vi "Main_12b.vi"() -> ()   [LabVIEW 2023]
uses:
  ENUM_Type.ctl
  <vilib>/Utility/error.llb/Trim Whitespace One-Sided.vi
panel:
  out "container size":i32
  out "appended array":T1[](array[typedef])
  out "Function Array min size":i32
  out "Array":cluster{"Array":T1[]}[](array[cluster])
  out "Rows Left":i32
  out "Complete Match Count":i32
  in  "Enum":T1
  out "Answer":i32
  in  "Puzzle":string="??#.????#???.#?# 1,5,1,1,1\n?##?##??#? 7,1\n??????#???. 1,7\n??#?#??#.?#.??#? 5,1,1,2\n???????.??? 1,3\n?#..##?##??###??#? 2,13\n?.????????.???????? 1,5,1,6\n?.???#???. 2,2\n??#..#???#? 1,1,4\n?.?##?????#??? 1,5,2,1\n.???#?????##??#.? 3,8\n?????????????.#.. 4,3,1\n..#???????.? 4,3,1\n????#??.?.#??? 7,3\n#??#???##??.?? 4,1,3,2\n??#?#?##?.???#??. 6,5\n???.#??.??###?.#?? 3,1,5,2\n?.????##??#?? 6,3\n???..?##????.? 2,3,1\n?.?#????.??#?#.? 1,2,1,3,1\n?.?###.???? 4,2\n?#???..??##? 4,3\n???#????#?. 1,2,3\n#???#???#??#???.? 1,10,1\n???????????????????? 1,5,6,3\n???????#??? 2,6\n??.??.????.?#?????# 1,1,2,1,4,3\n???#???.??#? 1,4,1,1\n???#???##??##? 3,2,3\n????.??????#?.#? 1,1,1,4,2\n?.#??#???? 1,1,5\n??##???#?.##??..? 4,2,4\n??????#.????.# 4,2,1,1\n??????#??#?.??? 2,7,1\n.????????##.?.?.##? 5,2,1,1,2\n.??????????#?#. 3,1,2,1\n?????????????. 2,1,5\n?##????#?.?????.#??? 2,1,2,3,3\n?????????#?.?????#? 1,2,1,3,4,2\n..?.#???.?##.? 1,3,2\n.??????????????? 10,2\n?.?#????#?.??? 1,1,2,2\n??????.#??.?.? 1,1,1\n#???#?#??#????? 1,2,1,5\n???.?.??#????.? 3,6\n.#.???###???.#?..??? 1,8,2,2\n.???.??#????# 2,4,1\n.????#?#?? 3,3,1\n?###??#??## 4,2,2\n??#?#???#???.??. 3,5,1\n???####??##..?#.#.?? 9,2,1,1\n??#?#???#.?. 5,1\n???#????#???##?# 2,3,3,1\n?#???????#???#??? 1,3,3,3,1\n#???#????#.##..? 8,1,2\n?????.?#?#??? 1,5\n.??#.??#?.? 1,1,1\n?#?#???#???.??? 1,1,4,1,3\n.????#.?.#??? 1,1,2,1\n.??#?.??#? 4,2\n#????????. 1,4,1\n??.#?#????#?...?? 1,8,2\n?#.#?#.??##? 2,3,1,2\n...??.?#?? 1,1\n?.?.????#..? 1,2,1\n?##????????.??.?#??? 6,1,1,4\n?.??#.??.?.???? 3,2\n.????.?????.???.?? 4,1,1,3,1\n?????????##???????#? 2,1,1,2,2,2\n???.?????.????? 2,3,5\n???#??????.??#??.? 1,6,1,1,1\n??##??????###??? 12,1\n?.??.?????? 1,1,2\n??#??????#?.. 2,5\n???#####????. 1,8\n.?#?##??????#??.???? 6,2,1\n?.#??#???????#????? 1,1,12,1\n??????????#.?..?##? 1,1,1,1,3,3\n???????#???.??## 10,4\n.?#????.?.???..? 1,1,2\n.???#?#????? 2,2,1\n#????#?.????##?#?# 1,5,1,5,1\n???.##??????##??#? 1,2,8,2\n??#????????????#? 6,7\n????.??.#.?#?#? 1,1,1,1,4\n??##?#??.#???? 6,1,4\n?#?.?#????????#?. 3,2,4,3\n..??????##?# 2,1,2,1\n?????????.???? 4,1,1,1\n.??#?????.?.?. 1,6,1\n#.?#?#??????#??# 1,6,2,1,1\n.#?.#.##??# 1,1,5\n??#?????#?????? 5,4\n.#??.?.?.? 2,1\n.?#???##.????##?? 7,2\n?#?.??????#??????# 1,8,3\n?.#??#??.?#.. 4,1,1\n?#?#?#??????? 7,1,1\n?#???????? 6,1\n????#..?#???##? 1,1,2,3\n..?????#?###??.? 1,9,1\n?##???.???#?# 4,4\n??.??#???..??#? 1,2,1,3\n#?#??????.??#?? 8,1,3\n???#?##?#?? 2,6\n.?.???#???.#?????? 1,3,1,5,1\n?#.???????# 2,2,1\n?.???.??.? 1,1,1\n?#?#?#??????#??#??? 1,5,2,4,2\n?#??.?#?????.?#. 4,6,2\n#???.?#?#??#?.??#? 2,7,1\n.??#...???????. 3,1,1\n?..???##??. 1,6\n??#??#?#??? 2,4\n?.?.??.??????#?. 1,7\n?.?????????.??. 2,2,2\n???.?????? 2,1\n???.??????????? 1,3,4,1\n?#????#???#??? 10,1\n??#???.?????#???# 6,3,1\n????.?##??#??# 3,8\n?????????????. 1,7,1\n?..?????.#???.. 1,4,2\n?.???#???#? 1,5,1\n#???.????? 2,1,1\n?#.??#?.???? 1,1,1,1\n????.?#???.???. 1,1,4,2\n.?#??#??.??????? 2,4,6\n.??.?##.??#?#.??? 2,3,2,1,1\n..??????#?.?? 2,2\n???#?#??.##. 3,2,2\n?..?????????##?#??? 1,13,1\n??#?????#?.??#?????? 6,2,5,2\n???.???#???# 1,1,3,1\n??##????.?. 4,1\n??#??#??#?. 3,6\n.??????#????#.#.?? 1,1,8,1,1\n?#?#?.?.?.###??#???? 5,1,1,3,1,1\n???.#?#???.?? 1,1,5,1\n?????####??????? 2,5,2,1\n????.??#??#? 1,1,2,1\n??.?????#?#.????? 2,3,3\n?#??#?#?.????.??? 2,3,2,2\n?????????#??.??????. 1,6,1,1,1,1\n???.##?##??#? 1,6,1\n????#?.??.. 4,1\n?#??#?#???.????#?# 4,4,6\n?????#??#.#? 1,2,2,1\n?#?#?#??###??? 1,1,7\n.##?.????? 3,3\n??#???###????? 1,6\n.?###????????##?#?? 7,1,5\n..?#????????#? 3,5\n#?#???.??? 1,1,1\n#???????????#??.??? 10,3,1\n???##??#??#?.?????. 10,3\n?#?????.???????## 3,2,5,3\n??.??#####???. 2,8\n???.?????? 1,1,3\n???#???????????. 6,4\n#???#?????##???.?#? 2,1,1,5,2\n?#?..???#??????. 2,7,2\n?????##?#? 2,3,2\n.#?..????# 2,3\n???????#??#.?..??.. 3,1,1,2,1,1\n?.#??#????? 1,3,2\n???..?.?.? 1,1,1\n?#.?#??#???.##.? 1,1,4,2\n???#?#.??#??? 4,1\n??????#????.???? 6,1,1,1,2\n???..??.#???? 1,1,1,2\n????????.? 1,1,1\n?..#??.??. 3,1\n?##.??#??? 2,1,1\n?????#?????#?#?? 2,12\n?#??????#???.?? 1,6,2,1\n#??.???.??##???.#? 2,3,7,2\n???????..????#????? 2,1,1,7,1\n????#??.?????? 1,2,4\n?###?#?##?##??.??. 12,1\n?#??#.?.??#?... 3,1,1,1,2\n??#??#??#????#? 9,2\n???????##????? 1,1,5\n?.?#????#?.??.?? 3,3,1,1\n???..??????#..??#? 1,1,7,1,1\n??.???###???#..? 1,1,5,1,1\n??.??.#????#????# 2,1,7,2\n??????#?#??????# 1,6,1\n#?.?...??.??????? 1,1,1,6\n??#?##??#?..## 7,2\n?#?###..?.#?##??.?.# 5,6,1\n.??.?.???. 2,1,1\n?.???..?.?#?.??.???? 1,3\n.#?.??????.?.?#??? 2,6,4\n???##...??. 3,1\n????????????#?????. 4,6\n????#.??#? 1,1,1\n?.?#.??..??#?????..? 1,2,1,8\n?????.??.? 1,2,1\n??????##?.?? 1,4\n???.????#??? 1,1,5\n.??#???.#.#??#??. 6,1,2,1,1\n?.????#??##?????? 1,1,1,7\n??????##.??? 3,2,1\n?.????#?????.?.? 1,4,2,1\n?????????????## 1,1,2,4\n.?##??#??.??# 4,1,3\n??#?##??#?? 2,5,1\n?????.###??.?.#??# 1,1,4,1,1,1\n.????????##?#? 1,7\n??????????.? 7,1\n.?????###????..#. 12,1\n????.????? 3,1,1\n#.??#????#????#????? 1,5,1,7,1\n.##??????.??##? 7,3\n?..?.???#?????###? 1,1,5,5\n??????#???. 1,1,3\n??.#???????##????. 1,2,3,6\n?.?.?.?.#???????#?. 1,1,1,1,2,7\n?????#????????. 1,1,1,4,1\n?.??#??#?? 1,1,2\n??#???.#.?#?#?? 1,1,1,1,5\n?????????.? 4,1\n??.?????#?.?.#?? 7,1\n??.?#.?????#??. 2,7\n?????##..? 1,4\n?????????. 4,1\n??.?..?#???? 2,3,2\n????.####??###? 2,4,4\n?####???##??????? 10,1,1\n???#?#???# 1,5,1\n????###.??.?????#??. 6,1,6\n#???????#?. 2,1,4\n?#?.???##???????#? 3,1,2,1,6\n???#??#?.?.?????? 1,5,1,1,4\n?.#???##???.?.## 1,3,2,2\n???..##?.?.? 2,2,1\n?.#?#?????. 3,1\n????.##?#?#??##?? 3,12\n#?##???????? 1,3,3,1\n???.#?.????##? 1,2,1,4\n???.??#???? 1,3\n.???###??.???????# 7,5,1\n?#.??.?#???##?. 1,1,1,4\n.????###????? 2,6\n???#???.???????#?? 1,2,1,3,4,1\n.?.?????????? 3,5\n??#???#?.###????.?? 7,3,1,1,1\n#??###??#?#.????? 11,1\n#.?????#??#.##???.? 1,1,7,5\n??????.????#???? 1,1,4,1,1\n?.?#?#?#??###?? 7,4\n????#???#?#?###????? 1,2,10,1\n????#????? 1,4,2\n???.#??#????.?#??.?. 3,2,1,1,4,1\n?????.?#??????. 1,2,1,1,1\n?#???????#?#?#???.? 2,12\n?#??..??.???###?? 4,2,1,5\n##????????#.? 5,2\n#?#?.?.??###??#?. 4,8\n??##?.???? 3,4\n?.????##???????? 8,1,1\n#????#??#???#?#.??? 15,1\n?.?????.#? 4,2\n?.##???..?? 1,3,1\n#????#??????????#?? 2,7,2,3\n???.????#? 1,1,2\n??..#?????### 1,3\n????????.?? 2,4,1\n#??##??#.?????.??? 1,5,2,1,1,1\n???#.?#?#?. 3,1,2\n?##?#??????#?#.# 3,3,3,1,1\n??.#?..??? 1,1,1\n?#??.???#? 1,1,3\n???#???????.??##?? 8,3\n??.#.?#???#??.? 2,1,7\n??????.####?.?#?# 4,4,4\n??????????? 2,2,1\n?#?.??.???.? 2,2\n????#?#?## 6,2\n.??###??????.? 5,3\n.???#.#????? 3,5\n?##?#?.?#?#??. 6,2,1,1\n#.???.??#?####?..? 1,1,1,8,1\n????#???#???# 1,1,2,3\n?????.??.#???#? 3,5\n?#??..?????????#?. 1,1,3,1,4\n#?????????????.?? 6,1,1,1\n?#?????..?????#??# 3,1,1,5\n???????.???????????? 1,4,1,9\n.????????????.. 2,1,6\n.?#??????. 2,4\n??#??#???#.???#? 1,5,2,1,2\n.?.???????.?.#??? 4,1,2\n##?.??##?..???. 3,4,3\n??..??#??#?. 1,6\n??#??????????##???? 2,6,4,1\n??..????##?????? 1,5\n##????????.??.#??? 2,6,4\n?#??#...?????# 2,2,1,2\n?..??????.???.?# 1,1,3,1,1\n.?###??#???#???? 7,4,1\n?#?.?????. 2,2\n??..????.?????# 1,1,2,2\n??##.#??????.##??#?? 1,2,1,1,1,5\n??.##??????#???#??? 4,8\n??#?????????. 4,3,2\n#????.???? 1,1,1\n?..??.?????? 2,3\n??????#??###???? 1,1,9,1\n?????#?#???????.. 1,6,3\n?#??.???#?##. 3,3,2\n?..##?#???????#?? 9,1\n???.?#?#?#?. 1,5\n???##?#???#?# 8,3\n?##??#??.??.???????? 2,3,1,6\n.??...?????????#.#? 1,6,2,2\n????.#??#?#.##?. 1,1,1,3,3\n?#?#?????.??????. 5,3\n??.????##???. 1,5\n????#?.???? 2,1\n????..??#???. 4,2,1\n???????.?# 2,1\n????????????? 1,1,3\n???##??????###.?#? 2,2,2,3,1\n??????#?#?#?#?## 3,10\n?????#??..????????? 8,5\n??##???????.??? 6,1,1,2\n?.???.????.??? 3,1,1,3\n.?.???.??? 1,2\n.???###???#??.?? 5,1,1,1\n????#?.##?###.# 1,3,2,3,1\n.?#???????? 1,4\n?#?#?????????### 8,6\n?????..???.???? 4,3,1,1\n..?#?.?#??? 1,5\n.????.??#? 3,3\n?##????.?#??????..?? 7,3,3,1\n?????##??.?.??...?? 9,2,2\n??..#??####??.?.?#? 8,2\n??????##????? 1,1,6\n??????#??.???#? 7,5\n???#..??.????. 4,1,2\n.#?.?###??? 1,4\n????###?...?#?#? 8,4\n?????#???#??????? 1,1,6,1,1\n.??#?#?##??????? 7,1,1\n.#.?????#.?#### 1,2,1,1,5\n?#??..#??.#?? 3,1,1,1\n????#??.???. 3,1,3\n#.???#???. 1,2\n???.???##.???.? 1,1,2,2\n?#?#..?#????##?.?. 3,9\n.?.??.????? 2,2\n??????.?.##?#?.? 5,4\n???#???.????? 7,1\n??####?????.???#?? 6,3,4\n?.?...?#.#?#??? 1,2,5\n??.??#??#?#?#??.?? 2,3,7,1\n?#?.???????? 1,1,1\n????????#?##?#??? 1,2,9,1\n#???.???#????.??#??? 3,1,1,1,4,1\n.??#?.?.#??? 2,1,2,1\n.?##?###.###?#?.??. 6,5,2\n.?.???????#????##? 3,10\n?.##???..#? 5,2\n????????????#??.???? 1,1,10,1\n??##??#.??#??#?? 5,3,2,1\n?#???#.??????..# 6,4,1,1\n????????.? 1,2,2\n?????#??#??#????#??? 14,2,1\n???#??.???#?#???? 4,7,1\n.?.##?.???#??..????? 1,3,4,2\n??????#??????? 1,1\n..#?##??.????. 5,3\n??????????#.? 4,1\n#????.???.? 1,1\n.?..?#.??? 2,1\n?#.??##??.##?.?? 2,4,2,2\n??#????#??????? 9,1\n.#?.##?##.#???? 1,5,1,1\n?#?###???#??#?.??? 11,1,1\n???#??..?? 3,1\n#?#??????#?????#? 12,2\n??#?#?.???.? 2,2,3,1\n?#???.?.??#?#???? 5,1,8\n.???#?#??#?????. 10,1\n??????.?????.? 5,1,1,1\n.?.??????????# 3,7\n.#?.??..##??.?#..#? 1,1,4,2,1\n?##?#??.??###?????# 2,1,1,1,7,1\n?##?.???.? 2,1,1\n?????#.#?##.?#? 1,1,4,1\n?#?.??.?#.#.##.? 2,1,1,1,2\n???????.#.??##??.?. 6,1,3,1,1\n.?#??#???????#???.#. 3,1,1,2,4,1\n?????#?.##??##??.?? 1,2,2,3,2\n#??.???????? 1,1,1,1\n????#?.##?.?#?#?# 5,2,5\n.?.??.#?????????..?# 1,1,6,1,2\n???#?#?????. 7,2\n???????##??#?.?#?.? 1,8,3\n.?..?#?#???? 4,1\n??.?#??.????. 1,1,3\n????##???##???#??? 12,4\n?###?#??..#?.??? 6,1,2,1\n##??..##?#????# 3,2,1,1\n?????#?##??##???#?? 2,13\n#?..???##???##?#???? 2,6,4,1,1\n.????.?....#????. 1,3\n?.?.??#??#.?# 1,2,1,2\n???#??.??#.? 1,1,1,2\n.????#?#???#??????? 12,1,1\n?..#??#?##??#???? 1,1,2,3,5\n.#??##?##??????.?# 2,11,2\n.?.#?#?.?#???#.? 1,4,6\n?#.##??.????? 2,4,4\n???.??????.??. 2,1,1,2\n???????.?##.#???.? 1,1,1,2,3,1\n??..???????#?.? 5,2\n?????#????? 3,2,2\n.##????..#??.. 6,2\n????.??????.???###? 3,3,1,5\n??????#?.???# 1,3,1,1\n????#????. 6,1\n??.?#????. 1,4\n??????#???##???. 6,1,3,1\n?.?#.????. 1,1,4\n?##??.#?#??.#?? 3,1,1,1,1\n?.?#??????. 1,5,1\n???????#?. 1,4\n???#????#?##?#?????? 2,2,1,1,6,1\n??##.?????##??#.? 1,2,7,1\n????????.# 4,1\n.???#????? 1,1,1\n?.?#??.????.?#?? 1,4,2,2,1\n.?##?#???.??..?#? 3,3,3\n?#??.?.?#??? 1,1,4\n????..#????#.?? 1,1,1,3,2\n???#?..??? 5,1\n?##???##.?. 3,2,1\n??#???.???### 2,1,1,3\n????.?#??##?. 2,2,2\n?#???##??#?????#.??? 2,11,1\n???#??..?##??# 5,6\n????.??#???.#?#.?#?# 2,5,1,1,1,1\n?.??????#??? 2,3,2\n#.#???..????????. 1,1,2,6,1\n?.?..?.#??????##?? 1,1,1,1,3,5\n.??.?.???? 1,1,4\n#??#.?#?#???#??????# 1,1,2,1,1,8\n?????.?#..#. 3,1,1\n????##???.?????.. 5,3\n.????#???????? 1,5,1,1\n##?..#.???#?????? 3,1,1,2,1\n#??##???????????. 1,11,1\n????????#. 2,1,2\n.#?#?????????. 1,4,2,1\n#??#??.????????????. 5,5,2\n..?#?#???#???????.?. 9,1,1,1\n?#?.?????????... 1,6\n??###??#?#?.? 5,2,1,1\n.?????????.??... 6,1\n?.?.#??#??????#?#. 1,2,7\n??.?#?.#??.??. 1,2,2,2\n?##?#.?#?. 3,1,1\n??.??####???... 2,6\n.?????#????..?..??## 7,1,3\n.#?##???.? 5,1\n?.?.???#.???. 1,1,2,1\n?????.???## 1,3,2\n.????#??.??.?. 5,1\n.?#??.???? 2,4\n??#?.??#?? 2,2\n?.??.??????.?????? 1,1,2,1,1,5\n?????#??????.??? 1,5,2\n#..?#??.?# 1,2,1\n???????#???#?#???.? 5,8\n??.?#??#?? 1,2\n????#.#??#? 3,1,1\n#?#?..?..?????#??? 4,1,2\n??????.?##?##.??? 1,4,6,1\n?.????###??? 1,8\n??##???????##?????. 8,4,1\n?#.?#.?.?????? 1,1,1,6\n???#?.?.#??##???##? 2,10\n.?????#?.?##????#?# 1,3,2,5\n#?.?.?#?..???#? 2,1,1,2,2\n..???#??.??#?? 5,3\n.????##??? 7,1\n??#?###???# 7,1\n?????????????????. 10,5\n??#?#?????????###?? 3,1,1,1,4,1\n????##???.#??? 1,6,1,1\n.##??????##?..??#?## 11,2,2\n?#.????????? 2,1,1,2\n??????#?.??#??..???. 3,1,5,3\n.?##??????????#???? 3,1,1,1,2,1\n?#?...?#?????#?.? 2,8\n###?#.#?#?????.#???? 5,1,2,2,4\n?.???#?#.?????#?.? 6,5\n#????#???#???#?#? 2,2,3,3\n??#??.??#.?#? 2,1,1,2\n##.?...????????#?#? 2,9\n??#?#???#???? 4,1,1,1\n.???#?.?????.?#?.#. 4,1,1,1,1\n??#.?????#?????##? 1,1,1,7\n#???????#?????#? 1,1,8\n????##?#?#??##???#?. 1,8,6\n#.???.?????.#?? 1,1,2,3\n##?????#??.????#? 2,1,3,6\n#???###?##.? 1,4,2\n#..??????#???.. 1,10\n?????#???.?#?#??# 7,7\n???.#????#?????.#? 1,1,1,6,1,1\n??.#?#?????????.?# 1,4,2,2,1\n?#?#?..?#? 1,2,2\n?.?##.???###?? 3,5\n.?#????#??..?? 2,5\n???#.#??.?.????..#?? 2,3,4,1,1\n???#..?????.? 1,1,5,1\n?##?#??????##? 4,1,5\n??#.#?###?##?????#? 1,1,8,1,1\n.#?#??#.#?.? 1,1,1,1\n????????#?#?##??# 5,1,1,5\n.??#?.?#?????.?????? 3,7,4\n?#?????#.?#? 2,5,2\n????.?#????#?????#? 1,9,2\n?#????#???.??.??.. 7,2,2\n?#.##???????.?#.? 2,5,1,2,1\n?.##?#?.????#?#??. 2,1,6\n?###??#.#????##.?? 5,1,1,1,3,1\n.??#?????#???#?.# 3,1,2,2,1\n?.????.??.#?????? 1,3,1,5,1\n????##?##?? 6,3\n.?#???.?.????? 2,1,4\n?????...??.. 1,1\n??#????..??# 1,2,2,3\n?###.?????#.???#? 4,3,1,2\n???##????.?#.?#??? 1,2,2,2,5\n?#.?????.?###?##??.? 2,5,6,1,1\n.????.??.?????????? 3,10\n??.?#?#.#..??? 1,3,1,1\n?.?#?#??.?. 5,1\n???#.?????##???#??? 2,13\n??#???#.#???#???#?? 2,2,11\n?#???????? 4,1\n??????##???##????# 2,10,1\n???#????#?? 3,1\n##????#.?.? 3,2\n.????#?????? 6,1\n?.??.????#? 1,4\n?????????.? 1,4\n#?#??#?##????#????#? 14,3\n#..#????#??? 1,1,4,1\n.?.##????.?? 1,2,1,2\n???.#??#?#?.?????? 1,1,7,1,1,1\n..?#????.#???##????? 3,2,7\n?????.??.? 3,1\n.?#??#?#..?#?.?##.?? 2,4,2,3,1\n???#?????.# 8,1\n????..##?.??#? 1,2,3\n.?????.?#? 1,1,1\n??#?.#?#?#?.###?. 1,5,4\n???.#????##.???##? 1,3,3,5\n?????????#?#?????? 7,2,1,1,1\n#.?##.???.?#?..?.#. 1,2,1,2,1,1\n???#.???.?? 1,1,3\n??.?.??###??.????.? 1,1,7,1,1,1\n.?.#.?#?##?.???# 1,1,5,1,1\n???###?#???# 8,2\n?.????.#..##??? 1,1,2,1,4\n??#????####???#?. 3,8\n#..?#????##?#?. 1,3,3,2\n###.??.##.? 3,1,2\n???##?.????#?#??? 4,5\n?.??.?.?.??? 1,1,1,1\n.#???##??#???##???? 1,1,5,4,1,1\n?..##..??#...?.?.?? 2,1\n?#..#???.?.??# 2,2,1,1\n????#?.#??.? 1,3,1,1\n?#?????#???.????? 3,3,1,2\n#.????###???.?#???? 1,7,2,2,2\n?????.?????? 3,1\n.??#???????. 3,1\n?.?#??.?#???##?#?? 1,1,1,11\n?#????#?#. 4,1,1\n..#?###???#.??? 1,7,2\n#....????? 1,1,1\n?.????????.? 4,1\n##?.??????.#??? 3,2,1,1,1\n?????.?#.?????#??.. 2,3\n?#??##?#?#?.??##? 7,2,3\n.?.?????##.??? 1,2\n.#?##?##?.?????.?#.. 7,1,1,2\n???..???#?. 1,1,2\n...?.???#?#? 1,4\n?????#????#.? 7,2\n??#????##???##. 3,2,4\n???.???????. 2,1,1,1\n###?..?????.. 3,4\n.???????????..?. 4,2,1\n?.?.#??.?? 1,1,1\n?????????????#?? 6,6\n..#?????.??? 4,1\n???#??#?##.?#?.?? 7,3\n#???###??????#?? 1,1,3,2,3\n?##??.??#??????#???# 3,9,1\n???#??#??.??????#??? 7,3,1\n.???###??##?#.?.??? 6,2,1,2\n?.?#?#?.?.?#? 3,2\n.??#.?###???##?? 2,5,3\n????.?????#??###?? 3,12\n?#?##?#..#??#?? 5,1,1,2\n??#??...???#?#???. 1,7\n???##???.???#.?. 7,3\n??.#???#.# 1,5,1\n??###???????????# 5,4,3\n#??..#??##.?????.? 1,1,5,2,1,1\n????#.???#????.. 3,4\n#?????.#??? 3,2,3\n?#?.???????. 2,2,2\n?.?????????## 1,1,4,3\n#????????..#?#????? 3,1,1,3,4\n???#??#??????????.. 7,1,1,2\n?##.??###???#?#??# 2,1,3,1,3,1\n?#?.???#?#?#?.??# 3,5,2\n??#????.??#?#? 3,3,4\n###?##???#?#??.?.# 8,3,1,1\n.??.?#???#??? 2,1,3\n.???#??###?? 1,6\n???????.???????? 7,1,2,1\n.??###?.??#.? 5,3\n?#???#???????#?#???? 2,5,1,4,2\n????.?????#?????? 1,1,7\n.??.?.?#?##?#???#?? 1,11\n?????#???? 5,2\n?.??.???.#?? 1,1,3\n????#???????? 5,3,1\n#?##????#???#?.?#.# 4,3,1,1,1\n??#??????#?? 1,1,1,4\n.????.#?????#?? 1,2,1,1,3\n????????????????? 1,4,3,2\n????.#?.##?##?#?#?? 3,1,5,3\n??#?###??? 1,3,1\n????#???....? 8,1\n.????.???.???..???. 2,3\n?????.??#? 4,2\n#??.#.????#.???###? 2,1,1,1,1,4\n.???????.??????# 6,5,1\n??#??#?????.??#. 1,4,1,2\n??#?.??.??????#?#??? 4,1,3,1,5\n?#??#???????#..??? 4,7,1\n???#?##?????.?? 5,2,1\n.?###?????#?##??. 6,7\n#??#..??????#?? 1,1,7\n.??#?#??????# 4,1,2\n.###??####????#???# 4,13\n????#?????.?. 6,1\n#?##???#????? 5,1,2\n??#?.##??????????? 4,4,5,1\n.????#???? 2,1,3\n?.?#.???????#?.????. 2,4,1,1,3\n?.?#?????##??????? 2,10,2\n?????..???##? 2,3\n?#.#.???#???.? 1,1,1,4\n.?##???##?????###??? 15,2\n?#.#?.????.??.?#?.? 1,2,3,1,1,1\n????#??????. 5,1\n?.#.????##??.?. 1,7\n??.?#?..??#?????.? 2,6\n???##?.#?.?#? 3,2,2\n?#?.???.?? 1,2\n?????????..?#??? 1,1,2,2,1\n?#.??..??? 1,1,2\n??.????##???? 1,1,3,1\n??####??????#.?.??? 5,1,1,1,1,1\n.??#????.?# 2,1,2\n..#?#???##???.?.??# 1,1,4,1,3\n??.##..??. 1,2,2\n?#???#?????? 2,5\n????##?#?.???.? 5,1\n.?#?..????#??.??? 1,4,1\n.#####??????#??. 7,5\n???.?.?.##?#???. 1,5\n????###??.????#?? 8,5\n?????#.???#?.?.?# 4,4,1,1\n????????.?###????#? 1,3,4,1,3\n?.?????.?#?????# 1,3,1,2,1\n??.??????????? 1,3,1,1\n???.?????#??? 1,6\n?##???#?#????#????#. 3,3,3,2\n??#?.?.???### 2,1,3\n#??..?##??????.??? 1,1,3,1,1,1\n???#??.?.#???#? 6,1,2\n?#?..????? 3,2\n?##??#???? 5,2\n??.??????.?#? 1,4,2\n.#?##???.???#??????? 7,4,1\n?.#???..????? 4,3\n.???..?#??##?? 1,7\n.#???????.??? 1,1,1,2\n?#?#???????##. 6,3\n#.?.#?????#??#?#???. 1,1,1,6,4,1\n.???????.?#?#??????? 2,5\n??.?.?????? 2,3\n???.????..#? 1,1,1,2\n??#??.?#?..???##??## 2,3,8\n#??.?.?#??#?. 2,5\n?.????.????????? 1,2,3,1,1\n???.??.??????????#. 1,1,1,3,3\n???????.??? 1,1\n##??#????????.?????# 2,2,6,1,3\n??.?????##????## 2,1,1,8\n???.??#?????#??.. 1,3,6\n??#?#??#???????.? 7,1\n.?#.????#??#? 2,4,2\n?????.??#.??? 1,2,2,1\n??##???.????????. 6,6\n..???..?.?.? 3,1\n??#?.??????.. 2,1\n???????##?????. 1,1,4,2,1\n??##..??#???. 2,4\n?????#??????#? 1,2,4\n..??#???#?????#?? 3,2,5\n???.??#??.???#?#??? 2,5,6,1\n?#?#.??##.?. 3,3\n#??#.?????.?? 4,2,1\n?#???.?#???#???.. 4,9\n????.??????#?#??# 2,7\n??#.??????????????? 3,7,5\n??#????###? 1,4\n???#????#.#.??.. 1,3,2,1,1\n???#?.???? 1,2\n?.??.?#??? 1,3\n??.????#??#.?.? 1,2,1,1,1\n..??????.?? 4,1\n??#?.???.???? 3,1,1,2\n?.????#????#? 4,3\n?#?????????????? 5,4,1,1\n?..?????#? 1,1,1\n?.?#???.?? 4,1\n#??#.????? 4,4\n#??.?????????????? 2,1,1,3,2,2\n.???#????.?? 1,1,2,1\n??.?##?.??#??#?#??.. 4,10\n????##????#???#.???? 2,3,2,1,1,1\n????????.??###?????? 7,5,2\n????.?.#??? 2,1,1\n.#?..?#????#???## 1,12\n#???##??.???????? 1,5,2,1,3\n???#???#?.#??..? 7,1\n?#????.???.?#? 6,2,1\n.#?????????#???. 6,1,3\n???###????????#?#?#? 8,2,1,4\n?#?#..??#???. 4,1,3\n.???##?#.??? 1,4,1\n??????????? 5,1,1\n??.#?#.???? 1,3,3\n.#.###??????.#? 1,4,1,1,1\n???#??.?.????? 1,3,4\n?#.#????????????# 1,1,1,8,1\n.??????###? 3,3\n.#???????#???? 3,1,4,1\n??#??.?#???#...? 3,6\n?#???????.?#???.???? 9,4,1,2\n???#.??#??? 4,3\n??#????#?#.??.?# 1,3,4,2\n????#?##?.??????? 6,1,2\n.??##?#?###..#??.?? 3,5,2\n??###???##?#?.??. 12,1\n?..#?????#????#?# 2,1,2,4\n????###?.?#??#??#. 8,6,1\n????##?#????# 10,1\n#?##?..?##?? 5,3\n?#.?#??#???????? 1,7,2,2\n.#?..?#?#??#. 2,6\n#??#????.??#?#. 7,3,1\n.?.??.????. 1,1,3\n?????.???#?#??.?? 1,3,4,1,2\n????????????#??#?? 4,8\n????####?#? 1,7\n?.#????.????#?.?? 1,6\n?#?????#?##?? 3,4\n?#????#????# 9,1\n?##?#?????.??? 6,1,1,1\n???..?##?..?????? 2,2,3\n#.??.??????? 1,1,2,1\n?##???##.?###? 3,2,4\n#?##????#.? 6,1,1\n.????.??###???#? 1,2,5,2\n?.#??.??#???? 1,3,4\n??##????#???#?#??? 4,7\n?#?.???#??##???#?? 1,1,2,8\n???.?#?##????.? 1,7\n#.?##?#?.#.????# 1,5,1,1,3\n#???..??#????#????? 4,5,2,1,1\n???????.???????#? 1,3,1,2,1\n##???????? 3,1\n?#..?.???? 1,1,1\n..??.#???##???#. 1,10\n.?????##?????#????. 7,4,1\n??..#?..#.#.#?. 1,2,1,1,2\n????.?###?#??. 2,8\n????.#?????? 3,6\n??#??#????#.?.?#.??. 10,2,2\n???#??????????? 8,2\n???.????#??..?. 1,5\n.?.??..?#. 1,1,1\n#??###..???#???? 6,1,1\n???###?..#?#??????? 5,7,1\n????#??#??#?#?.??#? 1,1,2,5,3\n????#??.?.?#???#. 7,1,1,1,1\n?##?#?#?.??#?. 6,1\n???????#?#???.# 1,4,1,1,1\n???????##.?# 9,1\n.?????#.???. 1,2,1,2\n#.?#.??#?? 1,1,1\n?##?#?????? 5,4\n?.?##??.#? 4,1\n?????##???.#?.##? 1,5,1,2\n??????.??? 1,1,2\n?.??.?#?#?#.?##??#?? 6,8\n??#???????????.?? 8,1\n#????????###??#??#? 1,2,8,1,2\n#.#???#?#?#.?????#? 1,9,1,1,1\n#.??#???##? 1,7\n?????##?????????#??? 6,1,2,4\n????#?##??????#?#?# 2,4,3,3\n?#?.##????#???? 1,3,2,1\n?.?.??#?.? 1,1,1\n???????#?#???..??? 1,4\n???.?#??##?#?##.#? 2,10,2\n??#?#???..???.??.? 7,1,1\n?????????.#.??????.? 6,2,1,1,3,1\n?#???##????# 2,6,1\n#?###?#??.#??..#.? 7,1,3,1,1\n???.???#???#?? 1,5,1\n??????#??????.???#? 7,4\n#?????#??.???#.? 3,3,1,1\n?.?..??.?##????.? 1,1,3,3\n?##????.???? 7,1,1\n?.?##.?#?#?????? 3,3,2\n?.??.?.??? 2,3\n?##?..????? 3,5\n??####?..?? 4,2\n???.???????????????. 1,7,6\n#???####???.# 8,1,1\n.#.???#?.????.? 1,2,3\n????????????#?????? 2,3,9,1\n#?#??#????????? 1,5,1,1,1\n.?.????.?#.?. 2,1\n????..#??? 1,1,1\n??##?????#???? 4,7\n?##?????.?#? 5,2\n???????###????##?# 3,1,6,2,1\n##?????.???. 4,2,2\n??#??.??#?..# 1,3,1\n????.#???????#?.. 1,10\n####??###????#.???. 5,3,3,3\n?#.?#???.?#? 1,4,3\n#.?#?#???#.#??????? 1,4,2,1,1,1\n??#????#?###???#?# 5,11\n??.???#???#????????? 1,5,3,1,2\n.??????#???####?.#?? 13,3\n.??????#?#?.??.?#? 10,1,2\n??..??##?#??????.??? 10,3\n????#???#####?????.. 10,2\n????#?#??#???###? 3,7\n????.#?.?????#.? 1,2,6\n???????????..? 1,4\n?.???#?????.? 1,2,1,1\n#??#??#?#???#?#.?? 1,8,3,2\n?????###????.???? 1,5,3\n???###?#?##????.??.? 1,9,1,1\n.?#?##???#????##??.. 9,3\n.?.?.?#????????##?. 1,1,1,1,1,4\n?.??.??#????##??##?? 3,6\n??????#?????.#?? 6,1,3\n?#?#???????.?#?.???. 11,3,1,1\n?.?#..#??????.??. 1,1,6,1\n??????#???### 3,8\n???#?#??.??##????#?? 8,1,8\n.#?.??.??#? 1,3\n?????.??????#?????. 2,1,1,10\n??.#????#.? 1,2,1\n???#?????????#?#?? 4,8\n..??..?????.### 1,2,3\n??.???#???.??# 1,7,1,1\n?###??..?.??#??#???? 5,4\n????????#?..?? 2,5,1\n???##?#?????#### 2,2,1,7\n?????#???#? 5,1,1\n??#.?#???####??#??.? 1,11,1\n?#?????##?#?? 5,5\n??.??.?####?. 1,6\n.???????#?????. 1,6,1\n????#.?????.??.?#? 1,1,1,2,1,2\n???.?#?????#.?#?.??? 1,4,1,1,2,3\n.#??????.#?? 1,1,1,1\n..#?.??????????? 2,5\n.??##???????. 3,4\n??#????#??????????.. 1,4,9\n.??#??.#.?# 2,1,1\n??.??????.?#????? 1,4\n#.?#??#???##? 1,2,7\n?###??.#.??. 4,1,1\n???#???#???. 7,1\n?????????#??? 4,4\n???.???????#.? 1,3,2\n?#??????##? 4,1,3\n?#.??.??#?.# 2,2,2,1\n?.#?????.????? 2,1,5\n?.#???#.?#?## 1,1,2,5\n#?#.?##???????#??.# 3,3,1,2,1\n#?#???.?.#.#??# 5,1,1,1,2\n??##?.##?????? 2,7\n.??###?#??#???? 5,1,6\n?.???#?????.?#??? 1,6,2\n??.?.?#??.???.???? 1,1,1,1,3,1\n???.???.###?##???## 1,1,1,6,3\n#???#??##??# 6,2,1\n??##??.##????? 3,7\n?#?#?#?.???##???.?#? 4,1,7,2\n.??#?#????.?##.? 8,2\n.???#???.. 1,1,1\n.????#??.#?#?. 2,4\n#?.?????????..?? 1,1,1,4,1\n?#???#??.? 1,2,1\n#???????????.???.? 4,3,1,1\n????#?#???#???#.?. 12,1\n???.??#.?#???#? 2,1,7\n??#?.#??.?#?. 1,1,2,1\n??#.???#.?? 2,2\n?????#??.????? 7,4\n?#?????????###?????. 1,1,1,1,5,2\n.?#?.#???? 2,3\n???###?#?..??.#?# 2,6,1,1,1\n..#?.???#?#???#??? 1,12\n????##.???? 3,2\n?#?????##?????? 1,2,5,1\n??????#???# 3,1,3\n.##??.???.? 3,1\n???##????...??..??? 6,2\n???????#???. 1,4,1\n?#??#???##?.??.# 10,2,1\n?.?.???#??? 1,1,3\n?#?#?#??..?? 8,1\n??#?.???????#?? 1,10\n?.#???#?#??????? 1,2,4,1,3\n#?#?.?##?????. 4,6\n#?#??.???#? 3,4\n?.?????#?#??. 1,8\n?.?.?.#.??.??#? 1,1,1,1,3\n?#???##??????##???.? 9,4,1\n?#???????????.? 5,1,1\n#???.??#?#????#?#? 2,1,11\n??#???????#???????? 6,1,7,1\n?#???#???????#?. 1,4,1,2\n????#??.???#.?? 6,2,1,1\n???.?#????.# 2,2,1,1\n#???#..??#?#????.? 5,7\n##?#..???.??.#?# 4,1,1,3\n.?..???????.????.?.. 2,3\n.???????.?? 4,1,1\n.?####??#?? 4,1\n??????#????#???? 1,1,6,3\n??#???#.????#??. 6,2,4\n?????????.#?? 5,2,2\n??#??..??????? 3,3\n.#?.??????#???. 1,2,1,1,1\n????????.?#????? 1,1,1,2,2\n?.??.??#??#?? 1,5\n.???#??????# 1,1,5\n?#?????.#?#?????? 2,1,1,3,5\n???#????#????#??#?## 1,1,4,2,5\n?.??.#.????..? 1,3\n??????#?#??? 8,1\n??#??.????#??.? 3,5\n?????#.?????#?#???.. 2,2,6\n????#.???. 1,1,1\n???#?.???#????# 1,2,9\n??#?#???###????#? 1,3,1,8\n#.???##??##? 1,1,2,2\n????#?????.#?.. 5,2\n..????.?????? 3,4\n????.??????? 2,1,2\n.?#??????????.? 7,2\n???#??????#?? 2,2,4,1\n???##?????#??#?. 1,9,2\n#????????.#??.? 1,3,1,1,1\n.??.#???#?##??.?? 1,2,2,4,2\n???.?????#. 1,2,2\n????#????.??? 5,1,1\n.????.??#?#?#???.? 3,5,3,1\n??????##??#.??? 1,2,5,1\n??????##.??.????.? 8,2,1\n?.?.?.?#?#?.????#?. 4,6\n..?????.?#??? 1,1,5\n???#?????????# 1,6,4"
  in  "Example":string="???.### 1,1,3\n.??..??...?##. 1,1,3\n?#?#?#?#?#?#?#? 1,3,1,6\n????.#...#... 4,1,1\n????.######..#####. 1,6,5\n?###???????? 3,2,1"
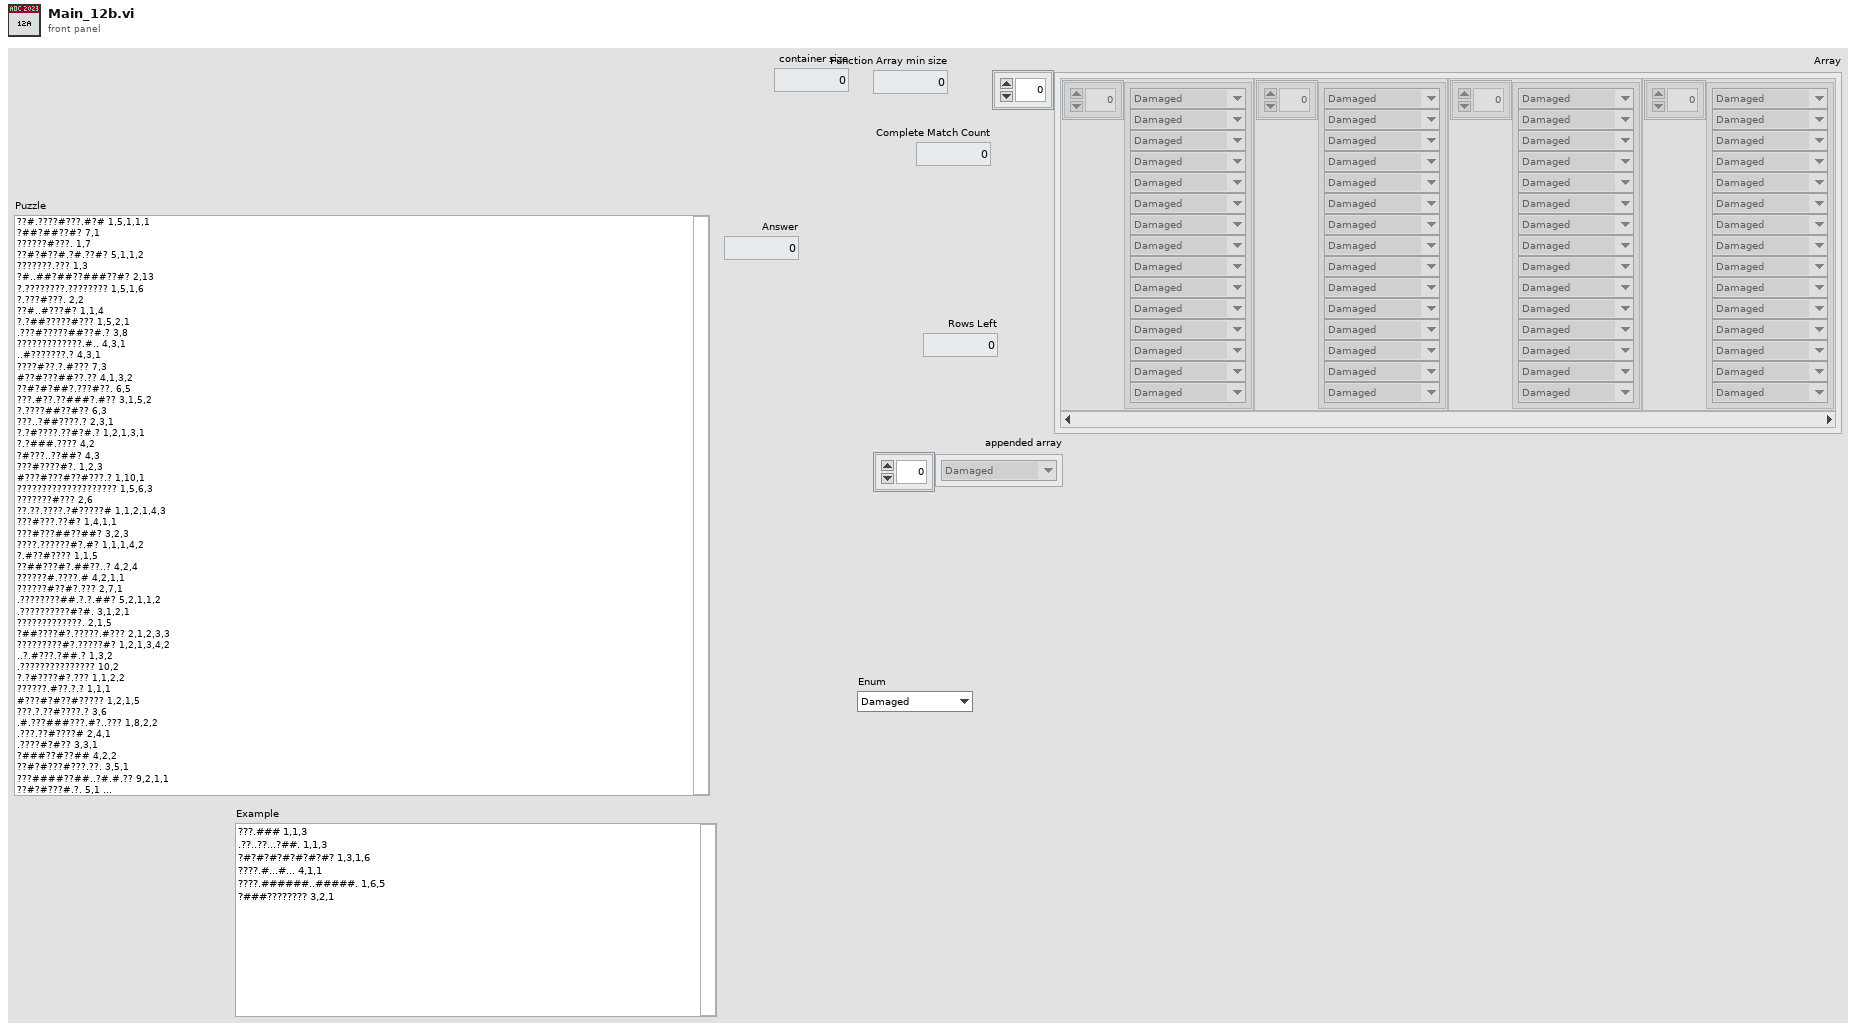
[diagram p1: front panel]
types:
  T1 = typedef "ENUM_Type.ctl" = enum16{"Damaged", "Operational", "Unknown"}
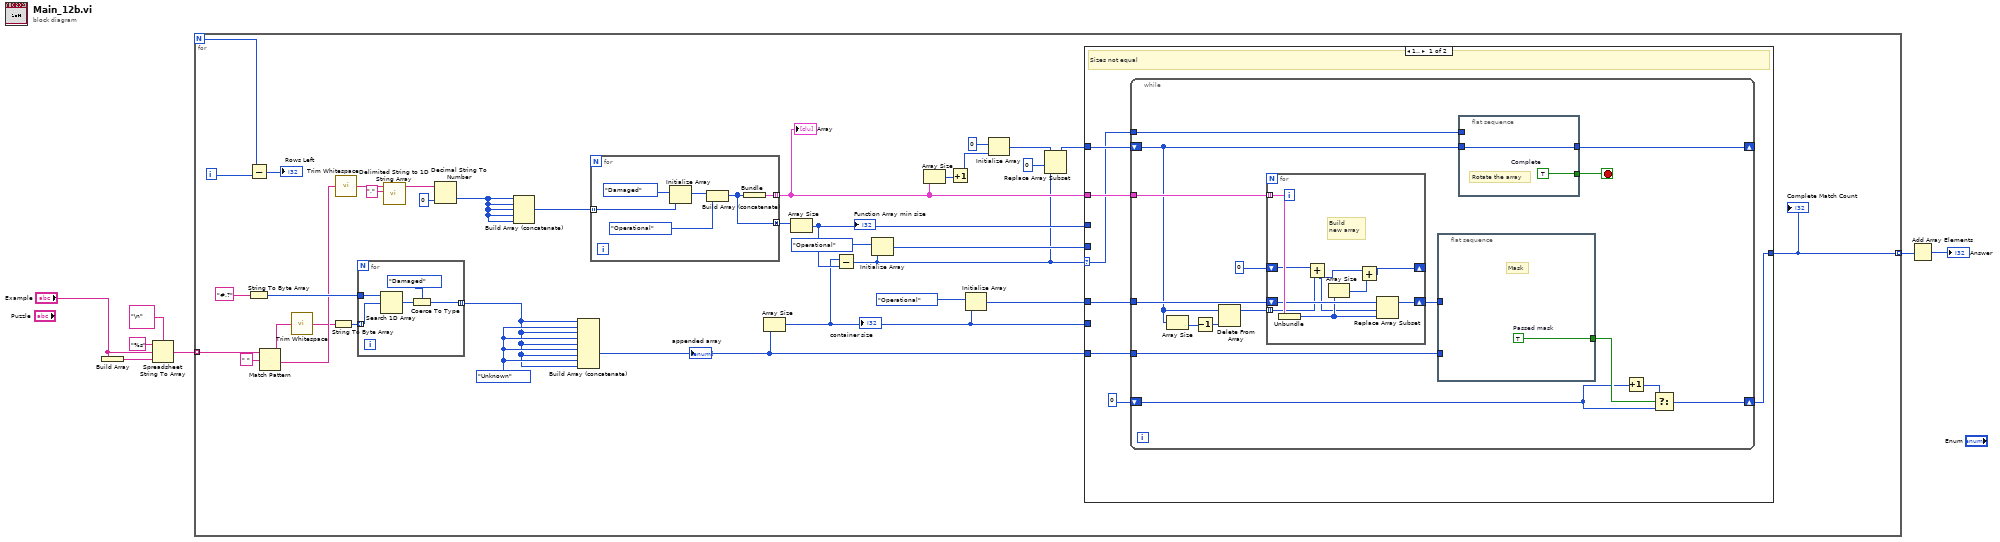
[diagram p0: block diagram]
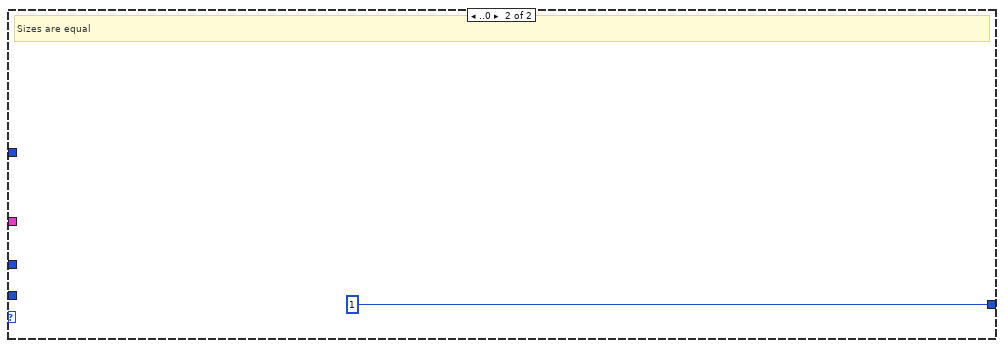
[diagram p2: hidden frame]
diagram:
  n1 = Build Array("Example") -> (w7:string[])
  n2 = Spreadsheet String To Array(delimiter (Tab)="\n", format string="%s", spreadsheet string="Example", array type (2D Dbl)=w7) -> (array=w4:string[])
  n3 = for {
    N -> [w28]
    tunnel: w4 -> [w43] mode=indexing
    tunnel: [w9] -> w2 mode=indexing
    i -> [w27]
    w31 = ENUM_Type."Unknown" ("Enum")
    n4 = Subtract(x=w28, y=w27) -> (x-y=→"Rows Left":i32)
    n5 = String To Byte Array(string="#.?") -> (unsigned byte array=w39:u8[])
    n6 = Match Pattern(string=w43, regular expression=" ") -> (before substring=w37:string, after substring=w38:string)  [unwired: 1 in, 2 out]
    n7 = call <vilib>:"Trim Whitespace.vi"("string"=w37) -> ("trimmed string"=w36:string)  [unwired: 1 in]
    n8 = String To Byte Array(string=w36) -> (unsigned byte array=w41:u8[])
    n9 = call <vilib>:"Trim Whitespace.vi"("string"=w38) -> ("trimmed string"=w35:string)  [unwired: 1 in]
    n10 = for {
      tunnel: w41 -> [w89] mode=indexing
      tunnel: w39 -> [w90]
      tunnel: [w86] -> w30 mode=indexing
      n11 = Search 1D Array(1D array=w90, element=w89) -> (index of element=w88:i32)  [unwired: 1 in]
      n12 = Coerce To Type(0:w88, 1:ENUM_Type."Damaged" ("Enum")) -> (2:w86:T1)
    }
    n13 = call <vilib>:"Delimited String to 1D String Array.vi"("delimiter"=",", "delimited string"=w35) -> ("string array"=w33:string[])  [unwired: 9 in]
    n14 = Decimal String To Number(string=w33, default (0L)=0 ("default (0 I32)")) -> (number=w29:i32[])  [unwired: 1 in, 1 out]
    n15 = Build Array (concatenate)(w29, w29, w29, w29, w29) -> (w25:i32[])
    n16 = Build Array (concatenate)(w30, w31, w30, w31, w30, w31, w30, w31, w30) -> (w23:T1[])
    "appended array" <- w23
    n17 = for {
      tunnel: w25 -> [w84] mode=indexing
      tunnel: [w81] -> w19 mode=indexing
      tunnel: [w80] -> w24 mode=concatenating
      n18 = Initialize Array(ENUM_Type."Damaged" ("Enum"), w84) -> (w83:T1[])
      n19 = Build Array (concatenate)(w83, ENUM_Type."Operational" ("Enum")) -> (w80:T1[])
      n20 = Bundle(w80) -> (w81:cluster{T1[]})  [unwired: 1 in]
    }
    "Array" <- w19
    n21 = Array Size(array=w23) -> (size(s)=w18:i32)
    "container size" <- w18
    n22 = Array Size(array=w24) -> (size(s)=w22:i32)
    "Function Array min size" <- w22
    n23 = Subtract(x=w18, y=w22) -> (x-y=w11:i32)
    n24 = Initialize Array(ENUM_Type."Operational" ("Enum"), w11) -> (w20:T1[])
    n25 = Array Size(array=w19) -> (size(s)=w10:i32)
    n26 = Increment(x=w10) -> (x+1=w8:i32)
    n27 = Initialize Array(ENUM_Type."Operational" ("Enum"), w18) -> (w16:T1[])
    n28 = Initialize Array(0 ("x-1"), w8) -> (w13:i32[])
    n29 = Replace Array Subset(array=w13, new element=w11, index=0) -> (w12:i32[])
    n30 = case shown="1.." w11 {
      selector: w11 -> [w44 _]
      tunnel: [w45 1] -> w9
      tunnel: w22 -> [_ _]
      tunnel: w23 -> [w47 _]
      tunnel: w19 -> [w50 _]
      tunnel: w18 -> [_ _]
      tunnel: w20 -> [_ _]
      tunnel: w16 -> [w49 _]
      tunnel: w12 -> [w48 _]
      frame 1.. {
        # "Sizes not equal"
        n31 = while {
          tunnel: w50 -> [w66]
          tunnel: w49 -> [w65]
          shift-right: [w64] -> _
          shift-left: w48 -> [w54]
          tunnel: w47 -> [w62]
          tunnel: w44 -> [w60]
          shift-right: [w56] -> w45
          shift-left: 0 ("size(s)") -> [w58]
          stop <- w61 stop-if-true
          n32 = Array Size(array=w54) -> (size(s)=w53:i32)
          n33 = Decrement(x=w53) -> (x-1=w52:i32)
          n34 = Delete From Array(array=w54, index=w52) -> (array with subset deleted=w55:i32[])  [unwired: 1 in, 1 out]
          n35 = for {
            tunnel: w66 -> [w78] mode=indexing
            tunnel: w55 -> [w74] mode=indexing
            shift-right: [w76] -> w63
            shift-left: w65 -> [w77]
            shift-right: [w70] -> _
            shift-left: 0 -> [w75]
            # "Build\nnew array"
            n36 = Unbundle(w78) -> (w72:T1[])
            n37 = Add(x=w75, y=w74) -> (x+y=w71:i32)
            n38 = Array Size(array=w72) -> (size(s)=w73:i32)
            n39 = Add(x=w71, y=w73) -> (x+y=w70:i32)
            n40 = Replace Array Subset(array=w77, new element=w72, index=w71) -> (w76:T1[])
          }
          n41 = flat-sequence {
            tunnel: w63 -> [_]
            tunnel: w62 -> [_]
            tunnel: [w67] -> w59
            frame #0 {
              w67 = TRUE  # Passed mask
              # "Mask"
            }
          }
          n42 = flat-sequence {
            tunnel: w54 -> [w69]
            tunnel: [w69] -> w64
            tunnel: [w68] -> w61
            tunnel: w60 -> [_]
            frame #0 {
              w68 = TRUE  # Complete
              # "Rotate the array"
            }
          }
          n43 = Increment(x=w58) -> (x+1=w57:i32)
          n44 = Select(t=w57, s=w59, f=w58) -> (s? t:f=w56:i32)
        }
      }
      frame ..0 {
        # "Sizes are equal"
      }
    }
    "Complete Match Count" <- w9
  }
  n45 = Add Array Elements(numeric array=w2) -> (sum=→"Answer":i32)
